vi "AnalyseResults.vi"(8 "error in (no error)":errorcluster, 11 "ResultArrayIn":T1 {"Time Stamp" format="%^<%.3X\n%x>T"}) -> (0 "error out":errorcluster, 1 "StringArray":string[][](array[string]), 2 "StatArray":dbl[][](array[numeric]), 3 "ResultArrayOut":T1 {"Time Stamp" format="%^<%.3X\n%x>T"})   [LabVIEW 2014]
uses:
  typedefs/ResultArray.ctl
  typedefs/Result.ctl
  typedefs/TVE_Fe_RFE.ctl
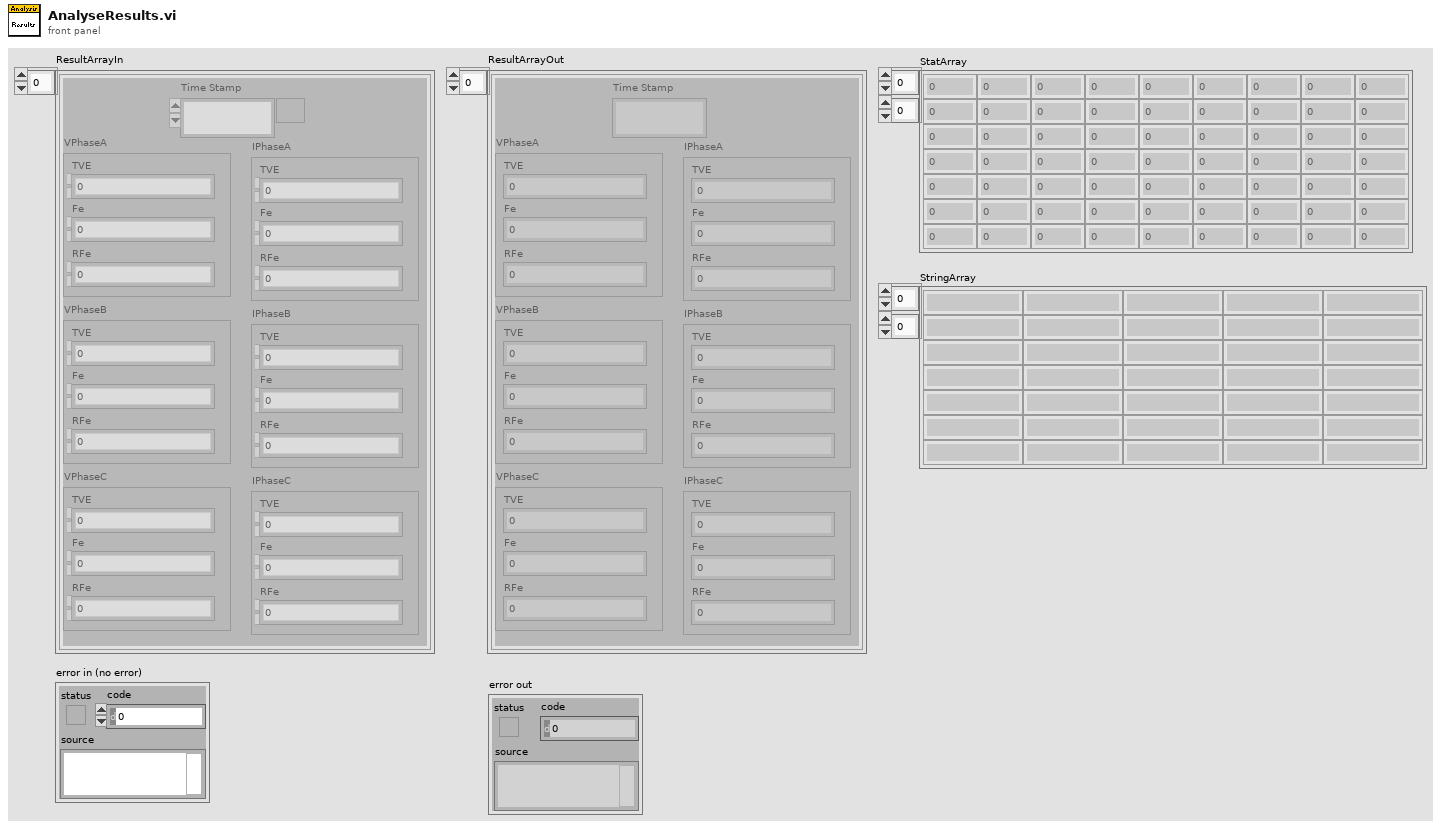
[diagram p1: front panel]
types:
  T1 = typedef "ResultArray.ctl" = T2[]
  T2 = typedef "Result.ctl" = cluster{"Time Stamp":timestamp, "VPhaseA":T3, "VPhaseB":T3, "VPhaseC":T3, "IPhaseA":T3, "IPhaseB":T3, "IPhaseC":T3}
  T3 = typedef "TVE_Fe_RFE.ctl" = cluster{"TVE":dbl, "Fe":dbl, "RFe":dbl}
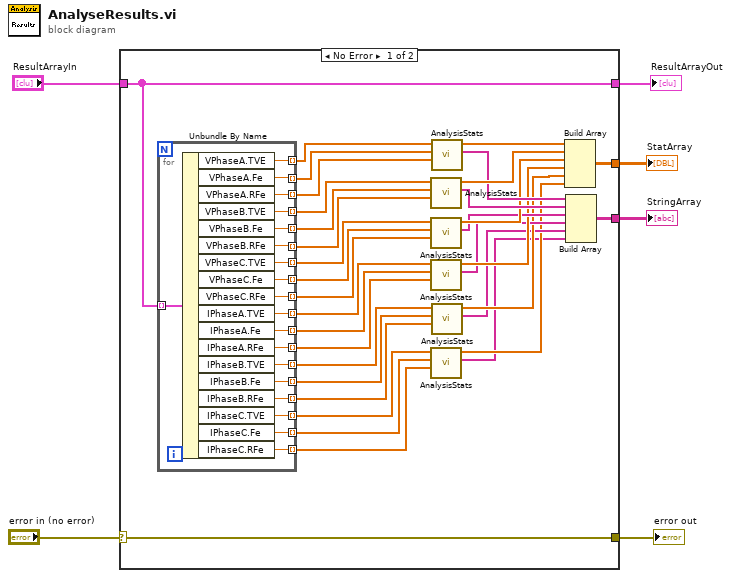
[diagram p0: block diagram]
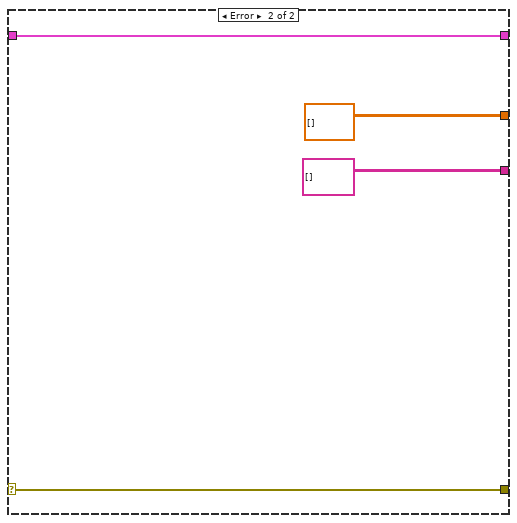
[diagram p2: hidden frame]
diagram:
  n1 = case shown="No Error" "error in (no error)" {
    selector: "error in (no error)" -> [w39 w63]
    tunnel: [w39 w63] -> w5
    tunnel: [w40 w62] -> w4
    tunnel: "ResultArrayIn" -> [w40 w62]
    tunnel: [w30 dbl[][] []] -> w2
    tunnel: [w27 string[][] []] -> w1
    frame No Error {
      n2 = for {
        tunnel: w40 -> [w59] mode=indexing
        tunnel: [w58] -> w38 mode=indexing
        tunnel: [w57] -> w37 mode=indexing
        tunnel: [w56] -> w36 mode=indexing
        tunnel: [w55] -> w35 mode=indexing
        tunnel: [w54] -> w34 mode=indexing
        tunnel: [w53] -> w33 mode=indexing
        tunnel: [w52] -> w26 mode=indexing
        tunnel: [w51] -> w25 mode=indexing
        tunnel: [w50] -> w24 mode=indexing
        tunnel: [w49] -> w21 mode=indexing
        tunnel: [w48] -> w20 mode=indexing
        tunnel: [w47] -> w19 mode=indexing
        tunnel: [w46] -> w16 mode=indexing
        tunnel: [w45] -> w15 mode=indexing
        tunnel: [w44] -> w14 mode=indexing
        tunnel: [w43] -> w11 mode=indexing
        tunnel: [w42] -> w10 mode=indexing
        tunnel: [w41] -> w9 mode=indexing
        n3 = Unbundle By Name(w59) -> ("VPhaseA.TVE"=w58:dbl, "VPhaseA.Fe"=w57:dbl, "VPhaseA.RFe"=w56:dbl, "VPhaseB.TVE"=w55:dbl, "VPhaseB.Fe"=w54:dbl, "VPhaseB.RFe"=w53:dbl, "VPhaseC.TVE"=w52:dbl, "VPhaseC.Fe"=w51:dbl, "VPhaseC.RFe"=w50:dbl, "IPhaseA.TVE"=w49:dbl, "IPhaseA.Fe"=w48:dbl, "IPhaseA.RFe"=w47:dbl, "IPhaseB.TVE"=w46:dbl, "IPhaseB.Fe"=w45:dbl, "IPhaseB.RFe"=w44:dbl, "IPhaseC.TVE"=w43:dbl, "IPhaseC.Fe"=w42:dbl, "IPhaseC.RFe"=w41:dbl)
      }
      n4 = call "AnalysisStats.vi"("RFeArray"=w33, "FeArray"=w34, "TVEArray"=w35) -> ("StringArray"=w28:string[], "StatArray"=w31:dbl[])  [unwired: 7 in]
      n5 = call "AnalysisStats.vi"("RFeArray"=w24, "FeArray"=w25, "TVEArray"=w26) -> ("StringArray"=w22:string[], "StatArray"=w23:dbl[])  [unwired: 7 in]
      n6 = call "AnalysisStats.vi"("RFeArray"=w19, "FeArray"=w20, "TVEArray"=w21) -> ("StringArray"=w17:string[], "StatArray"=w18:dbl[])  [unwired: 7 in]
      n7 = call "AnalysisStats.vi"("RFeArray"=w9, "FeArray"=w10, "TVEArray"=w11) -> ("StringArray"=w7:string[], "StatArray"=w8:dbl[])  [unwired: 7 in]
      n8 = call "AnalysisStats.vi"("RFeArray"=w36, "FeArray"=w37, "TVEArray"=w38) -> ("StringArray"=w29:string[], "StatArray"=w32:dbl[])  [unwired: 7 in]
      n9 = call "AnalysisStats.vi"("RFeArray"=w14, "FeArray"=w15, "TVEArray"=w16) -> ("StringArray"=w12:string[], "StatArray"=w13:dbl[])  [unwired: 7 in]
      n10 = Build Array(w32, w31, w23, w18, w13, w8) -> (w30:dbl[][])
      n11 = Build Array(w29, w28, w22, w17, w12, w7) -> (w27:string[][])
    }
    frame Error {
    }
  }
  "error out" <- w5
  "ResultArrayOut" <- w4
  "StatArray" <- w2
  "StringArray" <- w1
